vi "PyLoN_data1.vi"(6 "Exposure Time (s)":dbl=0.004 min=0.0 step=0.001 format="%.3f", 7 "Number of Images":u32=1 min=1 step=1, 8 "error in (no error)":errorcluster, 9 "PumpOffBkgd":dbl[](array[numeric]), 10 "PumpOnBkgd":dbl[](array[numeric]), 11 "Camera Handle":u32) -> (0 "error out":errorcluster, 1 "Pump_Off":dbl[](array[numeric]), 2 "Pump_On":dbl[](array[numeric]), 3 "Camera Handle 2":u32 caption="Camera Handle", 4 "Raman_Gain":dbl[](array[numeric]))   [LabVIEW 2014]
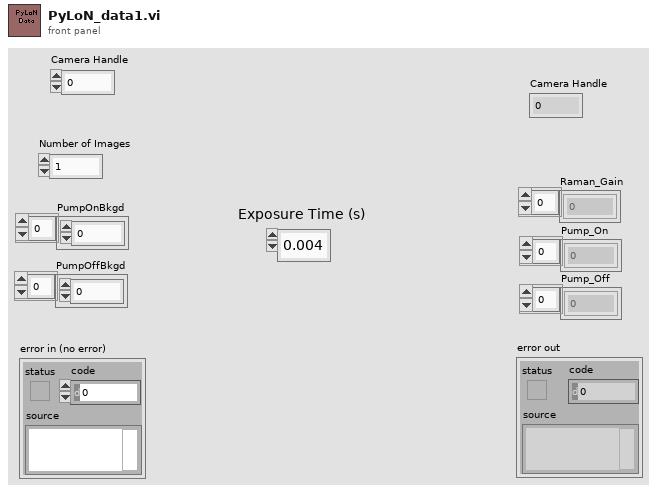
[diagram p1: front panel]
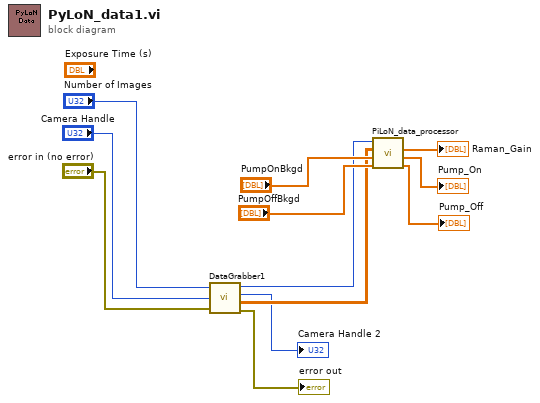
[diagram p0: block diagram]
diagram:
  n1 = call "DataGrabber1.vi"("# Images In"="Number of Images", "Camera Handle"="Camera Handle", "error in (no error)"="error in (no error)") -> ("# Images In"=w1:u16, "Camera Handle"=→"Camera Handle 2":u32, "Data"=w5:dbl[][], "error out"=→"error out":errorcluster)
  n2 = call "PiLoN_data_processor.vi"("PumpOffBkgd"="PumpOffBkgd", "PumpOnBkgd"="PumpOnBkgd", "Data"=w5, "# of Images"=w1) -> ("Pump_Off"=→"Pump_Off":dbl[], "Pump_On"=→"Pump_On":dbl[], "Raman_Gain"=→"Raman_Gain":dbl[])  [unwired: 5 in]
